vi "OP600ZP_Ubatt_Post_Relax.vi"(9 "errin":errorcluster caption="error out", 11 "Ubatt Post Relax":dbl) -> (1 "errout":errorcluster caption="error out", 3 "Dans la gamme ?":bool, 4 "MIN":dbl, 6 "MAX":dbl)   [LabVIEW 2020]
uses:
  VG/PackType.vi
  VG/IS30%.vi
  OP600ZP_VGConf.vi
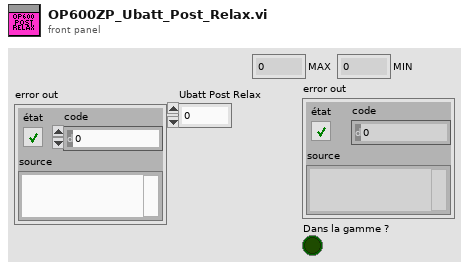
[diagram p1: front panel]
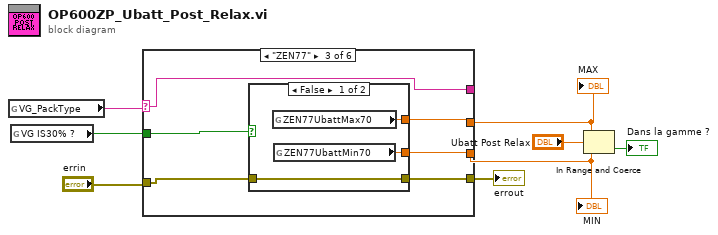
[diagram p0: block diagram]
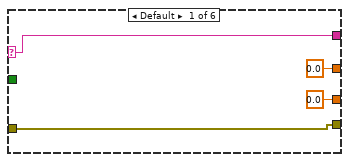
[diagram p2: hidden frame]
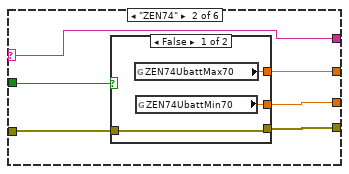
[diagram p3: hidden frame]
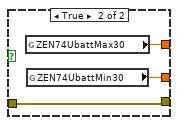
[diagram p4: hidden frame]
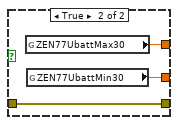
[diagram p5: hidden frame]
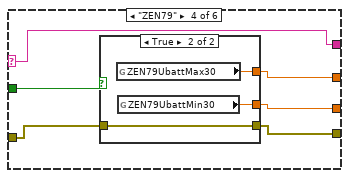
[diagram p6: hidden frame]
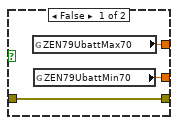
[diagram p7: hidden frame]
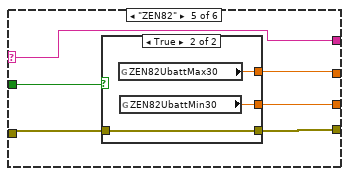
[diagram p8: hidden frame]
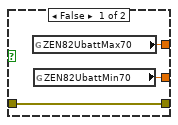
[diagram p9: hidden frame]
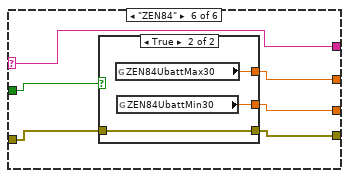
[diagram p10: hidden frame]
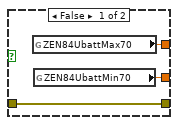
[diagram p11: hidden frame]
diagram:
  n1 = global read "PackType.vi" "VG_PackType"() -> (w8:string)
  n2 = global read "IS30%.vi" "VG IS30% ?"() -> (w5:bool)
  n3 = case shown="\"ZEN77\"" w8 {
    selector: w8 -> [w12 w15 w27 w39 w51 w63]
    tunnel: [0.0 ("ZEN84UbattMax30") w18 w30 w42 w54 w66] -> w6
    tunnel: [0.0 ("ZEN84UbattMin30") w17 w29 w41 w53 w65] -> w7
    tunnel: w5 -> [_ w16 w28 w40 w52 w64]
    tunnel: [w12 w15 w27 w39 w51 w63] -> _
    tunnel: "errin" -> [w11 w14 w26 w38 w50 w62]
    tunnel: [w11 w13 w25 w37 w49 w61] -> w3
    frame Default {
    }
    frame "ZEN74" {
      n4 = case shown="False" w16 {
        tunnel: [w21 w24] -> w18
        tunnel: [w20 w23] -> w17
        tunnel: [w19 w22] -> w13
        tunnel: w14 -> [w19 w22]
        frame False {
          n5 = global read "OP600ZP_VGConf.vi" "ZEN74UbattMax70"() -> (w21:dbl)
          n6 = global read "OP600ZP_VGConf.vi" "ZEN74UbattMin70"() -> (w20:dbl)
        }
        frame True {
          n7 = global read "OP600ZP_VGConf.vi" "ZEN74UbattMax30"() -> (w24:dbl)
          n8 = global read "OP600ZP_VGConf.vi" "ZEN74UbattMin30"() -> (w23:dbl)
        }
      }
    }
    frame "ZEN77" {
      n9 = case shown="False" w28 {
        tunnel: [w33 w36] -> w30
        tunnel: [w32 w35] -> w29
        tunnel: w26 -> [w31 w34]
        tunnel: [w31 w34] -> w25
        frame False {
          n10 = global read "OP600ZP_VGConf.vi" "ZEN77UbattMax70"() -> (w33:dbl)
          n11 = global read "OP600ZP_VGConf.vi" "ZEN77UbattMin70"() -> (w32:dbl)
        }
        frame True {
          n12 = global read "OP600ZP_VGConf.vi" "ZEN77UbattMax30"() -> (w36:dbl)
          n13 = global read "OP600ZP_VGConf.vi" "ZEN77UbattMin30"() -> (w35:dbl)
        }
      }
    }
    frame "ZEN79" {
      n14 = case shown="True" w40 {
        tunnel: [w45 w48] -> w42
        tunnel: [w44 w47] -> w41
        tunnel: w38 -> [w43 w46]
        tunnel: [w43 w46] -> w37
        frame False {
          n15 = global read "OP600ZP_VGConf.vi" "ZEN79UbattMax70"() -> (w45:dbl)
          n16 = global read "OP600ZP_VGConf.vi" "ZEN79UbattMin70"() -> (w44:dbl)
        }
        frame True {
          n17 = global read "OP600ZP_VGConf.vi" "ZEN79UbattMax30"() -> (w48:dbl)
          n18 = global read "OP600ZP_VGConf.vi" "ZEN79UbattMin30"() -> (w47:dbl)
        }
      }
    }
    frame "ZEN82" {
      n19 = case shown="True" w52 {
        tunnel: [w57 w60] -> w54
        tunnel: [w56 w59] -> w53
        tunnel: w50 -> [w55 w58]
        tunnel: [w55 w58] -> w49
        frame False {
          n20 = global read "OP600ZP_VGConf.vi" "ZEN82UbattMax70"() -> (w57:dbl)
          n21 = global read "OP600ZP_VGConf.vi" "ZEN82UbattMin70"() -> (w56:dbl)
        }
        frame True {
          n22 = global read "OP600ZP_VGConf.vi" "ZEN82UbattMax30"() -> (w60:dbl)
          n23 = global read "OP600ZP_VGConf.vi" "ZEN82UbattMin30"() -> (w59:dbl)
        }
      }
    }
    frame "ZEN84" {
      n24 = case shown="True" w64 {
        tunnel: [w69 w72] -> w66
        tunnel: [w68 w71] -> w65
        tunnel: w62 -> [w67 w70]
        tunnel: [w67 w70] -> w61
        frame False {
          n25 = global read "OP600ZP_VGConf.vi" "ZEN84UbattMax70"() -> (w69:dbl)
          n26 = global read "OP600ZP_VGConf.vi" "ZEN84UbattMin70"() -> (w68:dbl)
        }
        frame True {
          n27 = global read "OP600ZP_VGConf.vi" "ZEN84UbattMax30"() -> (w72:dbl)
          n28 = global read "OP600ZP_VGConf.vi" "ZEN84UbattMin30"() -> (w71:dbl)
        }
      }
    }
  }
  "errout" <- w3
  "MAX" <- w6
  "MIN" <- w7
  n29 = In Range and Coerce(upper limit=w6, x="Ubatt Post Relax", lower limit=w7) -> (In Range?=→"Dans la gamme ?":bool)  [unwired: 1 out]
